vi "Terminal.vi"(1 "Add":string, 2 "Head":string, 3 "LINE":i32) -> (0 "Str Out":string)   [LabVIEW 2015]
panel:
  out "all rows":i64[][](array[numeric])
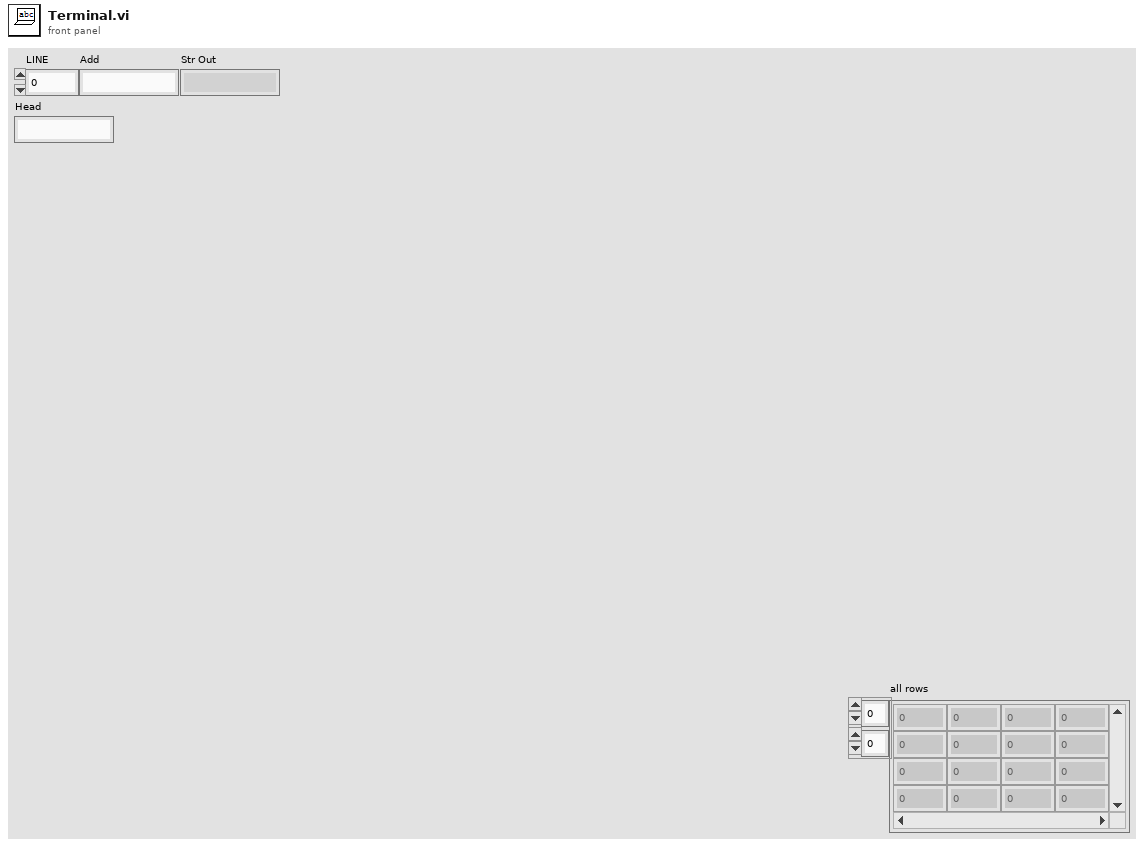
[diagram p1: front panel]
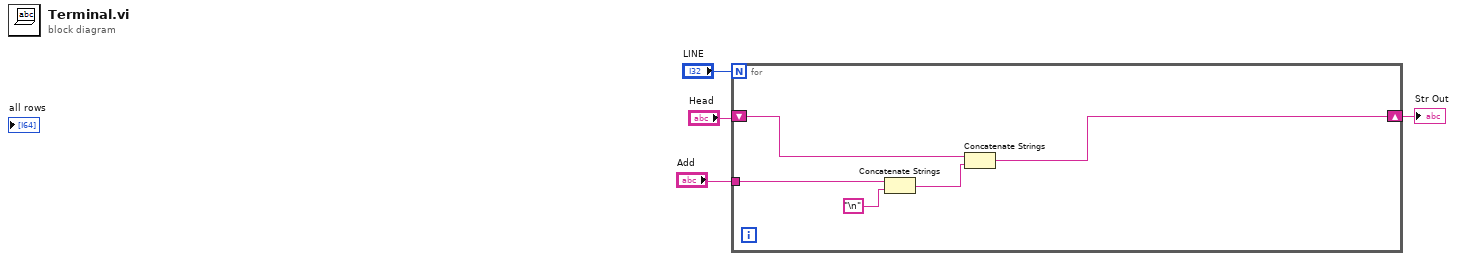
[diagram p0: block diagram]
diagram:
  n1 = for {
    N: "LINE" -> [_]
    shift-right: [w6] -> w1
    shift-left: "Head" -> [w7]
    tunnel: "Add" -> [w5]
    n2 = Concatenate Strings(w5, "\n") -> (w8:string)
    n3 = Concatenate Strings(w7, w8) -> (w6:string)
  }
  "Str Out" <- w1
